vi "UserInterface_ModuleQueue.vi"(7 "?":T5, 8 "error in (no error)":errorcluster, 11 "DataIn":T1) -> (0 "error out":errorcluster, 1 "Queue size":i32, 3 "queue out":refnum<queue>)   [LabVIEW 2020]
uses:
  Controller/#typedef_ControllerQueue_States.ctl
  #typedef_UserInterface_Data.ctl
  Cmd_enum.ctl
  #typedef_Parameters_cluster.ctl
  BaudRate_enum.ctl
panel:
  out "elements":T1[](array[typedef])
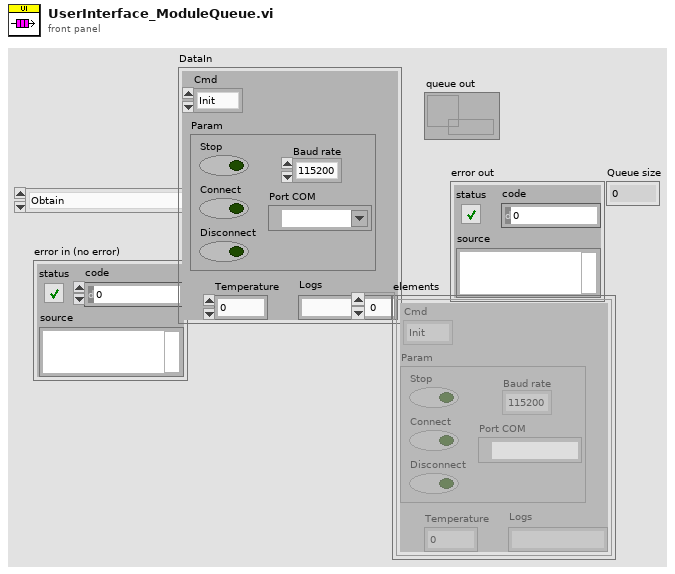
[diagram p1: front panel]
types:
  T1 = typedef "#typedef_UserInterface_Data.ctl" = cluster{"Cmd":T2, "Param":T3, "Temperature":dbl, "Logs":string}
  T2 = typedef "Cmd_enum.ctl" = enum16{"Init", "PrintChart", "Connect", "Disconnect", "ReadData", "Exit"}
  T3 = typedef "#typedef_Parameters_cluster.ctl" = cluster{"Stop":bool, "Connect":bool, "Disconnect":bool, "Port COM":refnum<visa-resource-name>, "Baud rate":T4}
  T4 = typedef "BaudRate_enum.ctl" = enum16{"115200", "9600"}
  T5 = typedef "#typedef_ControllerQueue_States.ctl" = enum16{"Obtain", "GetRef", "Enqueue", "EnqueueAtOpp", "GetStatus", "Flush", "Release"}
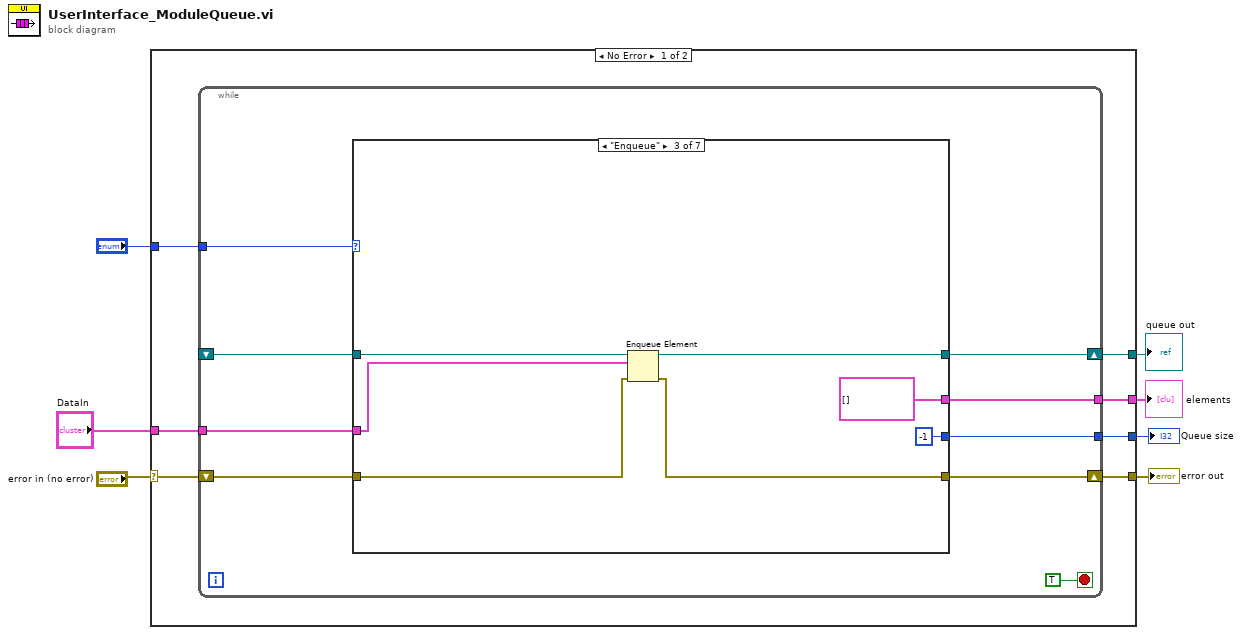
[diagram p0: block diagram]
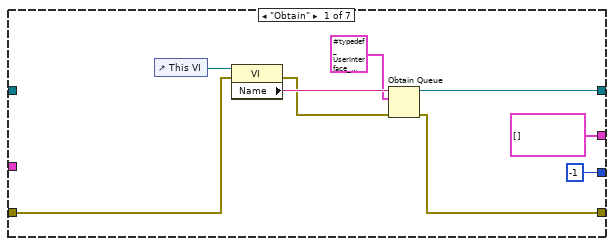
[diagram p2: hidden frame]
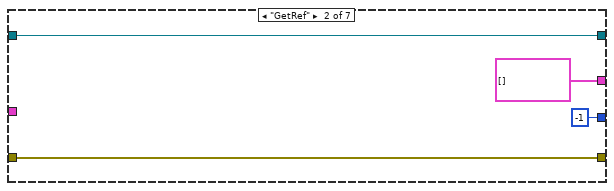
[diagram p3: hidden frame]
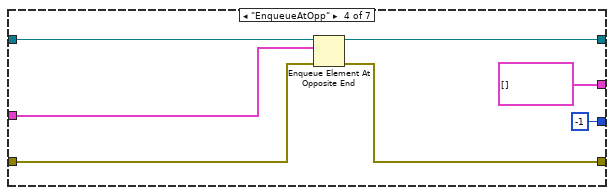
[diagram p4: hidden frame]
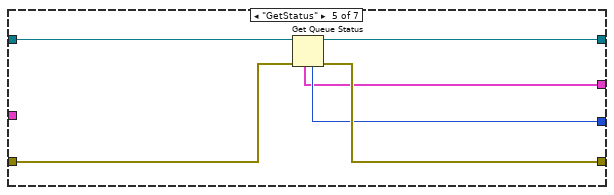
[diagram p5: hidden frame]
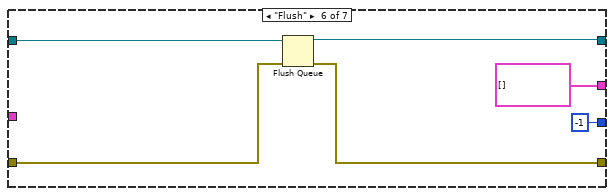
[diagram p6: hidden frame]
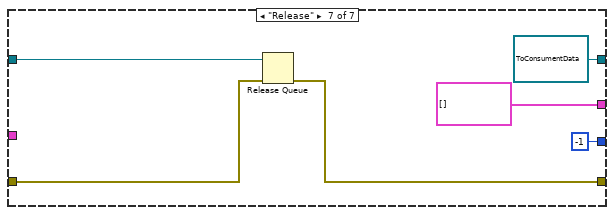
[diagram p7: hidden frame]
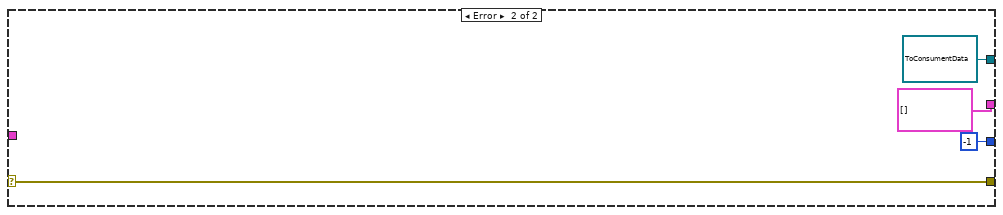
[diagram p8: hidden frame]
diagram:
  n1 = case shown="No Error" "error in (no error)" {
    selector: "error in (no error)" -> [w14 w72]
    tunnel: [w13 w72] -> w6
    tunnel: "?" -> [w12 _]
    tunnel: "DataIn" -> [w11 _]
    tunnel: [w10 -1 ("# elements in queue")] -> w4
    tunnel: [w9 refnum<queue> refnum ("queue out")] -> w1
    tunnel: [w8 T1[] [] ("elements")] -> w2
    frame No Error {
      n2 = while {
        shift-right: [w22] -> w13
        shift-left: w14 -> [w23]
        tunnel: w12 -> [w21]
        tunnel: w11 -> [w20]
        tunnel: [w18] -> w10
        shift-right: [w16] -> w9
        shift-left: _ -> [w17]
        tunnel: [w15] -> w8
        stop <- TRUE stop-if-true
        n3 = case shown="\"Enqueue\"" w21 {
          tunnel: w23 -> [w28 w35 w40 w47 w54 w60 w67]
          tunnel: [w31 w35 w41 w46 w53 w59 w66] -> w22
          tunnel: w20 -> [_ _ w38 w48 _ _ _]
          tunnel: [-1 -1 -1 -1 w52 -1 ("# elements in queue") -1 ("# elements in queue")] -> w18
          tunnel: [w25 w34 w42 w49 w55 w61 refnum<queue> refnum ("queue out")] -> w16
          tunnel: w17 -> [_ w34 w43 w50 w56 w62 w68]
          tunnel: [T1[] [] ("elements") T1[] [] ("elements") T1[] [] ("elements") T1[] [] ("elements") w51 T1[] [] ("elements") T1[] [] ("elements")] -> w15
          frame "Obtain" {
            n4 = control-ref of="This VI"() -> (w30:refnum<vi>)
            n5 = property class="VI"(reference=w30, error in=w28) -> (error out=w27:errorcluster, "Name"=w29:string)  [unwired: 1 out]
            n6 = Obtain Queue(name (unnamed)=w29, element data type=T1 {"Cmd"=enum."Init", "Param"={"Stop"=FALSE, "Connect"=FALSE, "Disconnect"=FALSE, "Port COM"="", "Baud rate"=enum."115200"}, "Temperature"=0.0, "Logs"=""} ("ToConsumentData"), error in (no error)=w27) -> (queue out=w25:refnum<queue>, error out=w31:errorcluster)  [unwired: 2 in, 1 out]
          }
          frame "GetRef" {
          }
          frame "Enqueue" {
            n7 = Enqueue Element(queue=w43, element=w38, error in (no error)=w40) -> (queue out=w42:refnum<queue>, error out=w41:errorcluster)  [unwired: 1 in, 1 out]
          }
          frame "EnqueueAtOpp" {
            n8 = Enqueue Element At Opposite End(queue=w50, element=w48, error in (no error)=w47) -> (queue out=w49:refnum<queue>, error out=w46:errorcluster)  [unwired: 1 in, 1 out]
          }
          frame "GetStatus" {
            n9 = Get Queue Status(queue=w56, error in (no error)=w54) -> (queue out=w55:refnum<queue>, error out=w53:errorcluster, # elements in queue=w52:i32, elements=w51:T1[])  [unwired: 1 in, 4 out]
          }
          frame "Flush" {
            n10 = Flush Queue(queue=w62, error in (no error)=w60) -> (queue out=w61:refnum<queue>, error out=w59:errorcluster)  [unwired: 1 out]
          }
          frame "Release" {
            n11 = Release Queue(queue=w68, error in (no error)=w67) -> (error out=w66:errorcluster)  [unwired: 1 in, 2 out]
          }
        }
      }
    }
    frame Error {
    }
  }
  "error out" <- w6
  "Queue size" <- w4
  "elements" <- w2
  "queue out" <- w1
